vi "Labview_code_used_to_design_external_transceiver.vi"() -> ()   [LabVIEW 2018]
doc: "Example: Stream to Disk\n\nRecommended Input Signal: 100kHz, 2Vpp, sine wave\n\nDevices Supported: Refer to NI Example Finder\n\nLabVIEW Description:\n\nThis example demonstrates streaming a continuous acquisition to disk. It configures and starts one acquisition that is never triggered. This is accomplished by configuring a software trigger and never sending the software trigger. Therefore, the digitizer will continuously acquire data into its onboard memory until Abort or Close is called. \n\nThe loop continuously fetches data from onboard memory and streams it to a binary file. If the sampling rate is low, the computer can fetch all the data from the digitizer, so data is never overwritten. However, at faster sampling rates, the computer will not be able to fetch the data before it is overwritten by new data. This results in the \"data overwritten\" error.\n\nThe input parameters to the Fetch VI include the maximum waveform size to fetch. Since a timeout of zero is set, the digitizer will return however many points are currently available rather than waiting for the requested number of samples. The Fetch VI will return a waveform with the actual number of points fetched. \n\nThe \"relative to\" property determines which samples to fetch from memory. In this example, it is set to the read pointer, which starts at the beginning of the acquisition and is incremented by the actual number of points during each fetch."
uses:
  Control 1.ctl
  <vilib>/Utility/error.llb/DialogType.ctl
  <instrlib>/niScope/Controls/niScope input clock source.ctl
  <instrlib>/niScope/Controls/niScope exportable signals.ctl
  <instrlib>/niScope/Controls/niScope export destinations.ctl
  <instrlib>/niScope/Controls/niScope trigger source digital.ctl
  <vilib>/Analysis/3filter.llb/Filter Passband Type.ctl
  <vilib>/DAQmx/write.llb/DAQmx Write (Digital Wfm 1Chan NSamp).vi
  <vilib>/DAQmx/create/channels.llb/DAQmx Create Channel (DO-Digital Output).vi
  <instrlib>/niScope/Configure/Trigger/niScope Configure Trigger Digital.vi
  <vilib>/DAQmx/configure/timing.llb/DAQmx Timing (Sample Clock).vi
  <vilib>/DAQmx/configure/trigger.llb/DAQmx Start Trigger (Digital Edge).vi
  <vilib>/Waveform/DWDTOps.llb/DWDT Boolean Array to Digital.vi
  <vilib>/Waveform/DWDTOps.llb/DWDT Append Digital Signals.vi
  <vilib>/Waveform/DWDTOps.llb/DWDT Uncompress Digital.vi
  <vilib>/DAQmx/miscellaneous.llb/DAQmx Fill In Error Info.vi
  <instrlib>/niScope/Acquire/Fetch/niScope Fetch Binary 16.vi
  <vilib>/Analysis/3filter.llb/Butterworth Filter (DBL).vi
  <vilib>/measure/maresamp.llb/Resample Waveform (single shot).vi
  <vilib>/Analysis/3filter.llb/FIR Filter (DBL).vi
  <resource>/objmgr/daqmx.rc
  <vilib>/measure/NI_MAPro.lvlib
  <vilib>/Analysis/NI_AAL_SigProc.lvlib
  <vilib>/Analysis/NI_AALBase.lvlib
panel:
  out "x-y":i32
  out "Mod. depth":dbl
  out "Threshold 2":dbl
  out "Threshold 1":dbl
  out "index of element 2":i32
  out "index of element":i32
  out "Peak - Valley":dbl[](graph) caption="Peak - Valley vs. Sample Number"
  out "# of peaks":i32
  out "Resampled data":waveform(dbl)(graph) caption="Signal vs. Time"
  out "Peak det. output":bool[](array[boolean])
  in  "Sample rate":dbl=2000000.0 caption="Digital Output Frequency" step=1000000.0 format="%.3p"
  out "Acquisition Complete":bool=TRUE
  out "Digital Waveform":digitalwaveform(graph)
  in  "Line(s)":tag="PXI1Slot5/port0/line1:3"
  in  "stop":bool
  out "Total Acquired Data (bytes)":i64 format="%.0p"
  in  "Total Samples to Acquire":u64=10000000 step=1048576 format="%.3p"
  in  "Continues data acquisition":bool=TRUE caption="Plot Data?"
  out "Memory per Channel":dbl format="%#_4p"
  out "Measurement Time (min)":dbl format="%.2f"
  out "Samples Used Onboard Memory":dbl(slide)=3898016.0 scale=-1.0..33554432.0 scale format="%.1p"
  out "Status":string="Acquisition in progress."
  out "Actual sample rate":dbl caption="Actual Sample Rate" format="%.3p"
  in  "Enforce realtime":bool=TRUE caption="Enforce Realtime"
  in  "Input Impedance":u32(ring) items=["1 mega ohm", "75 ohms", "50 ohms"]
  in  "Channel BW":T1=5000000.0 format="%.1p"
  in  "Channel":string="0" caption="Channel Name(s)"
  out "Format":string
  in  "Confirm File Replace?":bool
  in  "File path":path=path "C:/Users/trial.txt"
  out "error out":errorcluster {"code" format="%.0x"}
  out "Last Points Fetched":i32=50000 format="%.3p"
  out "Total Points Fetched":i64 format="%.0p"
  in  "resource name":refnum<k15>="PXI1Slot3" caption="Resource Name"
  in  "Max Points Per Fetch":u32=55000 format="%.3p"
  in  "Min sample rate":dbl=20000000.0 caption="Min Sample Rate" step=1000000.0 format="%.3p"
  in  "vertical range":dbl=2.4 caption="Vertical Range" format="%.2f"
  # "Vertical and Horizontal"
  # "Settings"
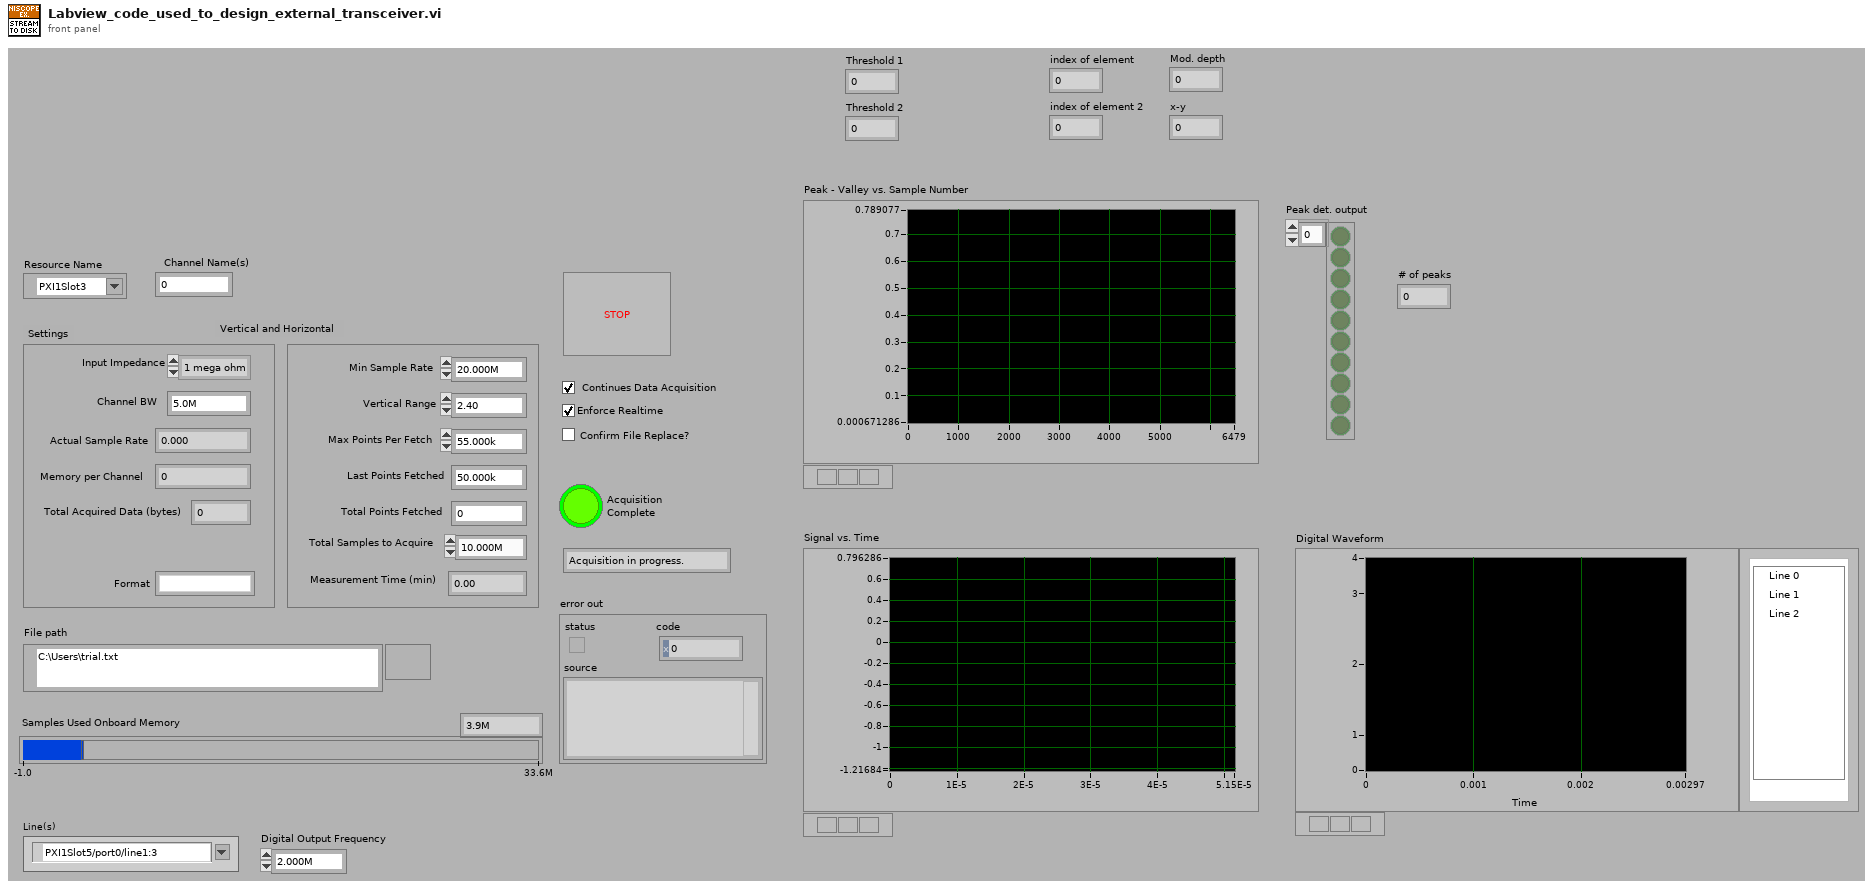
[diagram p1: front panel]
types:
  T1 = typedef "Control 1.ctl" = dbl
  T2 = typedef "niScope trigger source digital.ctl" = string
  T3 = typedef "niScope export destinations.ctl" = string
  T4 = typedef "niScope exportable signals.ctl" = u16
  T5 = typedef "niScope input clock source.ctl" = u16
  T6 = typedef "DialogType.ctl" = u16
  T7 = enum16{"open", "open or create", "create or replace", "create", "open (read only)"}
  T8 = typedef "NI_AALBase.lvlib/Filter Passband Type.ctl" = enum32{"Lowpass", "Highpass", "Bandpass", "Bandstop"}
  T9 = cluster{"alias rejection (dB)":dbl, "normalized bandwidth":dbl}
  T10 = cluster{"actualSamples":i32, "absoluteInitialX":dbl, "relativeInitialX":dbl, "xIncrement":dbl, "offset":dbl, "gain":dbl, "reserved1":dbl, "reserved2":dbl}
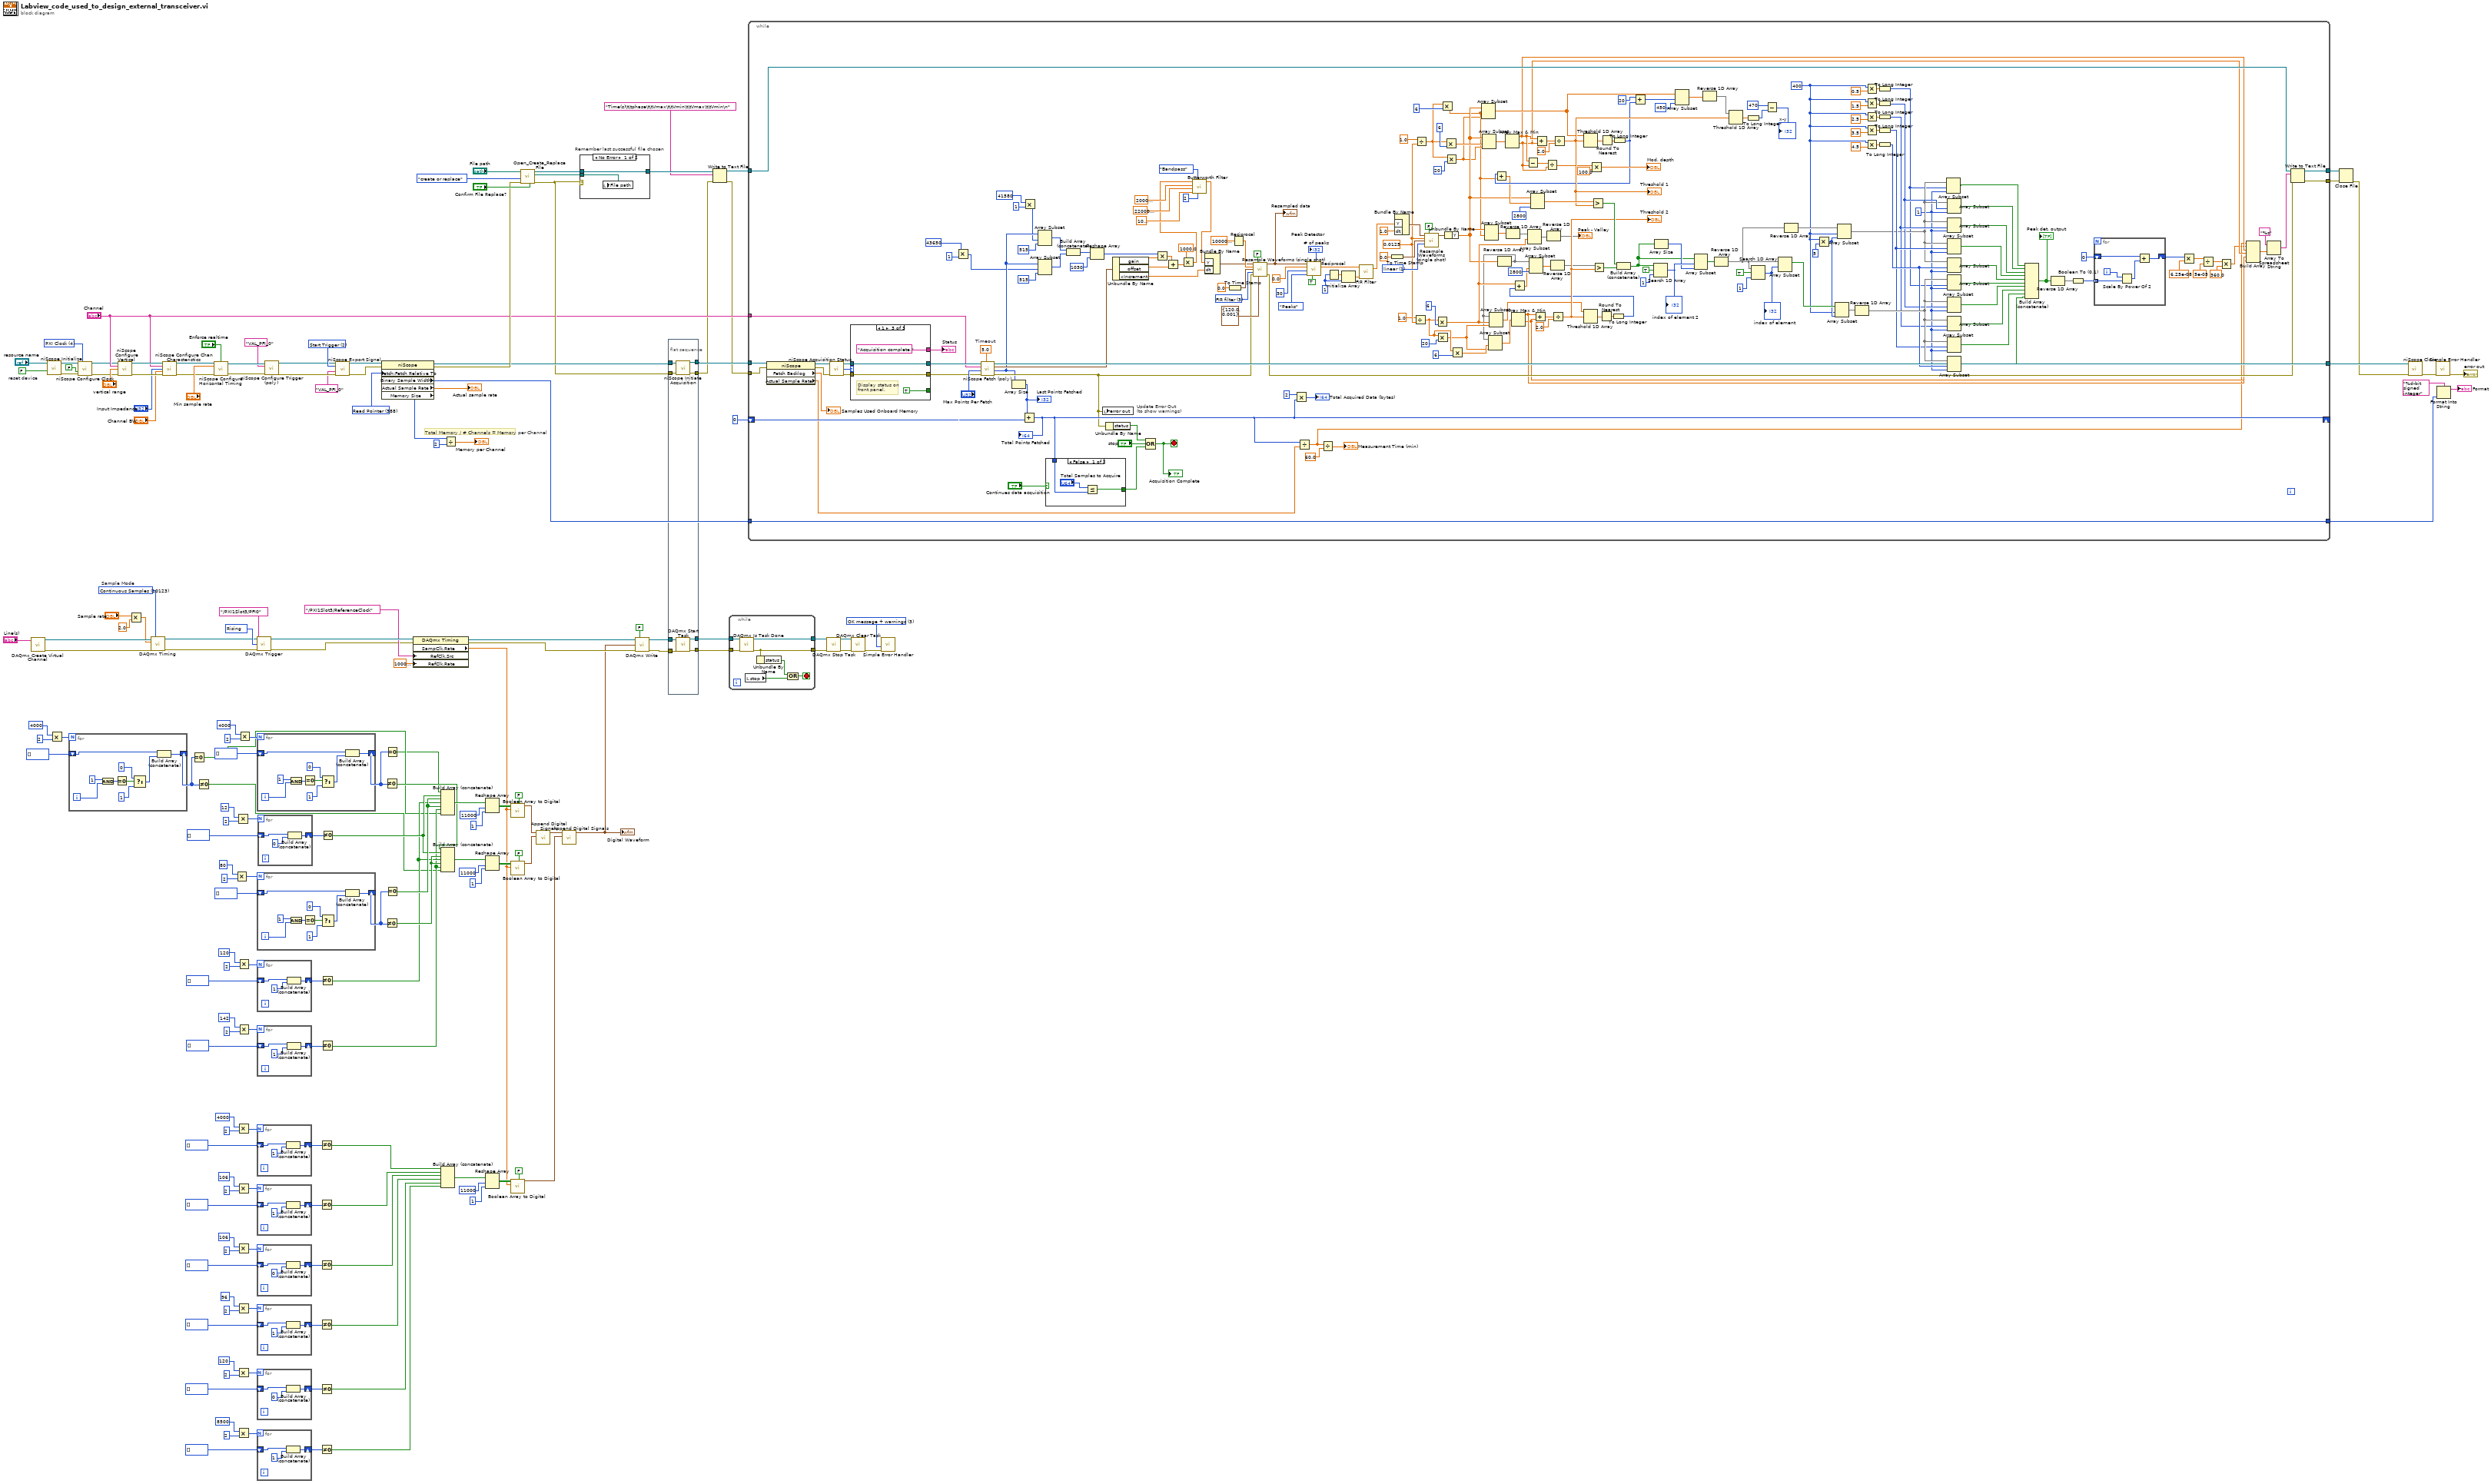
[diagram p0: block diagram]
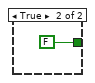
[diagram p3: hidden frame]
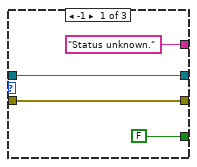
[diagram p4: hidden frame]
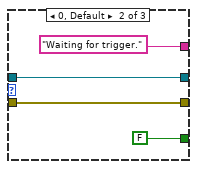
[diagram p5: hidden frame]
diagram:
  w132 = 10280 items=["Rising"=10280, "Falling"=10171] ("edge")
  w137 = T4 2 items=["None"=0, "Start Trigger"=2, "Advance Trigger"=5, "Reference Trigger"=1, "End of Record Event"=4, "End of Acquisition Event"=3, "Ready for Start Event"=7, "Ready for Advance Event"=6, "Ready for Reference Event"=10, "Reference Clock"=100, "Sample Clock"=101, "5 Volt Power"=13] ("signal")
  w142 = 10123 items=["Finite Samples"=10178, "Continuous Samples"=10123, "Hardware Timed Single Point"=12522]  # Sample Mode
  w143 = T5 4 items=["None"=0, "RTSI Clock"=1, "PFI 0"=6, "PFI 1"=2, "PFI 2"=3, "PXI Clock"=4, "External"=5, "Clock In"=7] ("input clock source")
  w151 = T6 3 items=["no dialog", "OK message", "continue or stop message", "OK message + warnings", "continue/stop + warnings"] ("type of dialog (OK msg:1)")
  w163 = 388 items=["Start"=482, "Trigger"=483, "Pretrigger"=477, "Now"=481, "Read Pointer"=388] ("Fetch:Fetch Relative To")
  w181 = FALSE  # reset device
  # "Total Memory / # Channels = Memory per Channel"
  # "Remember last successful file chosen"
  n1 = call-poly <vilib>:"DAQmx Create Virtual Channel.vi"("lines"="Line(s)") -> ("task out"=w66:refnum<k21>, "error out"=w65:errorcluster)  [unwired: 13 in]
  n2 = call <instrlib>:"niScope Initialize.vi"("resource name"="resource name", "reset device"=w181) -> ("instrument handle"=w150:refnum<k15>, "error out"=w149:errorcluster)  [unwired: 12 in]
  n3 = Multiply(x=4000, y=2) -> (x*y=w8:i32)
  n4 = for {
    N: w8 -> [_]
    shift-right: [w189] -> w3
    shift-left: i32[] [] -> [w190]
    i -> [w186]
    n5 = And(x=1, y=w186) -> (x .and. y?=w187:i32)
    n6 = Equal To 0?(x=w187) -> (x = 0?=w185:bool)
    n7 = Select(t=0, s=w185, f=1) -> (s? t:f=w182:i32)
    n8 = Build Array (concatenate)(w190, w182) -> (w189:i32[])
  }
  n9 = call <instrlib>:"niScope Configure Clock.vi"("instrument handle"=w150, "input clock source"=w143, "master enabled"=FALSE, "error in"=w149) -> ("instrument handle out"=w72:refnum<k15>, "error out"=w71:errorcluster)  [unwired: 10 in]
  n10 = call <instrlib>:"niScope Configure Vertical.vi"("instrument handle"=w72, "channels"="Channel", "vertical range"="vertical range", "error in"=w71) -> ("instrument handle out"=w168:refnum<k15>, "error out"=w167:errorcluster)  [unwired: 10 in]
  n11 = Multiply(x="Sample rate", y=2.0) -> (x*y=w63:dbl)
  n12 = call-poly <vilib>:"DAQmx Timing.vi"("task/channels in"=w66, "sample mode"=w142, "rate"=w63, "error in"=w65) -> ("task out"=w130:refnum<k21>, "error out"=w129:errorcluster)  [unwired: 10 in]
  n13 = call <instrlib>:"niScope Configure Chan Characteristics.vi"("instrument handle"=w168, "channels"="Channel", "input impedance"="Input Impedance", "maximum input frequency"="Channel BW", "error in"=w167) -> ("instrument handle out"=w68:refnum<k15>, "error out"=w67:errorcluster)  [unwired: 9 out]
  n14 = Equal To 0?(x=w3) -> (x = 0?=w2:bool[])
  n15 = Not Equal To 0?(x=w3) -> (x != 0?=w5:bool[])
  n16 = call <instrlib>:"niScope Configure Horizontal Timing.vi"("instrument handle"=w68, "enforce realtime"="Enforce realtime", "min sample rate"="Min sample rate", "error in"=w67) -> ("instrument handle out"=w135:refnum<k15>, "error out"=w134:errorcluster)  [unwired: 10 in]
  n17 = Multiply(x=80, y=2) -> (x*y=w92:i32)
  n18 = Multiply(x=12, y=2) -> (x*y=w95:i32)
  n19 = Multiply(x=4000, y=2) -> (x*y=w50:i32)
  n20 = Multiply(x=106, y=2) -> (x*y=w45:i32)
  n21 = Multiply(x=106, y=2) -> (x*y=w40:i32)
  n22 = Multiply(x=96, y=2) -> (x*y=w35:i32)
  n23 = Multiply(x=120, y=2) -> (x*y=w19:i32)
  n24 = Multiply(x=8500, y=2) -> (x*y=w12:i32)
  n25 = Multiply(x=120, y=2) -> (x*y=w89:i32)
  n26 = Multiply(x=142, y=2) -> (x*y=w24:i32)
  n27 = Multiply(x=4000, y=2) -> (x*y=w100:i32)
  n28 = call-poly <vilib>:"DAQmx Trigger.vi"("task/channels in"=w130, "source"=tag "/PXI1Slot3/PFI0", "edge"=w132, "error in"=w129) -> ("task out"=w128:refnum<k21>, "error out"=w69:errorcluster)  [unwired: 10 in]
  n29 = for {
    N: w50 -> [_]
    shift-right: [w191] -> w53
    shift-left: i32[] [] -> [w193]
    n30 = Build Array (concatenate)(w193, 1 ("element")) -> (w191:i32[])
  }
  n31 = for {
    N: w45 -> [_]
    shift-right: [w194] -> w48
    shift-left: i32[] [] -> [w196]
    n32 = Build Array (concatenate)(w196, 1 ("element")) -> (w194:i32[])
  }
  n33 = for {
    N: w40 -> [_]
    shift-right: [w197] -> w43
    shift-left: i32[] [] -> [w199]
    n34 = Build Array (concatenate)(w199, 0 ("element")) -> (w197:i32[])
  }
  n35 = for {
    N: w35 -> [_]
    shift-right: [w200] -> w38
    shift-left: i32[] [] -> [w202]
    n36 = Build Array (concatenate)(w202, 1 ("element")) -> (w200:i32[])
  }
  n37 = for {
    N: w19 -> [_]
    shift-right: [w203] -> w21
    shift-left: i32[] [] -> [w205]
    n38 = Build Array (concatenate)(w205, 0 ("element")) -> (w203:i32[])
  }
  n39 = for {
    N: w12 -> [_]
    shift-right: [w206] -> w15
    shift-left: i32[] [] -> [w208]
    n40 = Build Array (concatenate)(w208, 1 ("element")) -> (w206:i32[])
  }
  n41 = for {
    N: w100 -> [_]
    shift-right: [w216] -> w107
    shift-left: i32[] [] -> [w217]
    i -> [w213]
    n42 = And(x=1, y=w213) -> (x .and. y?=w214:i32)
    n43 = Equal To 0?(x=w214) -> (x = 0?=w212:bool)
    n44 = Select(t=0, s=w212, f=1) -> (s? t:f=w209:i32)
    n45 = Build Array (concatenate)(w217, w209) -> (w216:i32[])
  }
  n46 = for {
    N: w92 -> [_]
    shift-right: [w225] -> w105
    shift-left: i32[] [] -> [w226]
    i -> [w222]
    n47 = And(x=1, y=w222) -> (x .and. y?=w223:i32)
    n48 = Equal To 0?(x=w223) -> (x = 0?=w221:bool)
    n49 = Select(t=0, s=w221, f=1) -> (s? t:f=w218:i32)
    n50 = Build Array (concatenate)(w226, w218) -> (w225:i32[])
  }
  n51 = for {
    N: w89 -> [_]
    shift-right: [w227] -> w101
    shift-left: i32[] [] -> [w229]
    n52 = Build Array (concatenate)(w229, 1 ("element")) -> (w227:i32[])
  }
  n53 = for {
    N: w24 -> [_]
    shift-right: [w230] -> w27
    shift-left: i32[] [] -> [w232]
    n54 = Build Array (concatenate)(w232, 1 ("element")) -> (w230:i32[])
  }
  n55 = for {
    N: w95 -> [_]
    shift-right: [w233] -> w103
    shift-left: i32[] [] -> [w235]
    n56 = Build Array (concatenate)(w235, 0 ("element")) -> (w233:i32[])
  }
  n57 = call-poly <instrlib>:"niScope Configure Trigger (poly).vi"("instrument handle"=w135, "trigger source"=T2 "VAL_PFI_0", "error in"=w134) -> ("instrument handle out"=w118:refnum<k15>, "error out"=w138:errorcluster)  [unwired: 11 in]
  n58 = Not Equal To 0?(x=w53) -> (x != 0?=w31:bool[])
  n59 = Not Equal To 0?(x=w48) -> (x != 0?=w34:bool[])
  n60 = Not Equal To 0?(x=w43) -> (x != 0?=w32:bool[])
  n61 = Not Equal To 0?(x=w38) -> (x != 0?=w33:bool[])
  n62 = Not Equal To 0?(x=w21) -> (x != 0?=w17:bool[])
  n63 = Not Equal To 0?(x=w15) -> (x != 0?=w11:bool[])
  n64 = Not Equal To 0?(x=w101) -> (x != 0?=w81:bool[])
  n65 = Not Equal To 0?(x=w27) -> (x != 0?=w23:bool[])
  n66 = Not Equal To 0?(x=w103) -> (x != 0?=w83:bool[])
  n67 = call <instrlib>:"niScope Export Signal.vi"("instrument handle"=w118, "signal"=w137, "output terminal"=T3 "VAL_PFI_0", "error in"=w138) -> ("instrument handle out"=w119:refnum<k15>, "error out"=w117:errorcluster)  [unwired: 10 in]
  n68 = property class="niScope"(reference=w119, error in=w117, "Fetch:Fetch Relative To"=w163) -> (reference out=w125:refnum<k15>, error out=w161:errorcluster, "Binary Sample Width"=w158:i32, "Actual Sample Rate"=→"Actual sample rate":dbl, "Memory Size"=w159:i32)
  n69 = Not Equal To 0?(x=w107) -> (x != 0?=w4:bool[])
  n70 = Not Equal To 0?(x=w105) -> (x != 0?=w82:bool[])
  n71 = Equal To 0?(x=w107) -> (x = 0?=w1:bool[])
  n72 = Equal To 0?(x=w105) -> (x = 0?=w84:bool[])
  n73 = property class="DAQmx Timing"(reference=w128, error in=w69, "RefClk.Src"=tag "/PXI1Slot3/ReferenceClock" ("source"), "RefClk.Rate"=10000000.0 ("SampClk.Timebase.Rate")) -> (reference out=w127:refnum<k21>, error out=w126:errorcluster, "SampClk.Rate"=w30:dbl)
  n74 = Build Array (concatenate)(w1, w83, w84, w81, w84, w23, w2) -> (w73:bool[])
  n75 = Build Array (concatenate)(w4, w83, w82, w81, w82, w23, w5) -> (w78:bool[])
  n76 = Build Array (concatenate)(w31, w34, w32, w33, w17, w11) -> (w59:bool[])
  n77 = Divide(x=w159, y=2) -> (x/y=→"Memory per Channel":dbl)
  n78 = Reshape Array(w73, 11000 ("dimension size"), 1 ("dimension size")) -> (w85:bool[][])
  n79 = Reshape Array(w78, 11000 ("dimension size"), 1 ("dimension size")) -> (w76:bool[][])
  n80 = Reshape Array(w59, 11000 ("dimension size"), 1 ("dimension size")) -> (w57:bool[][])
  n81 = call-poly <vilib>:"Boolean Array to Digital.vi"("compress data (F)"=FALSE, "sample rate"=w30, "boolean array"=w85) -> ("digital waveform"=w75:digitalwaveform)  [unwired: 7 in, 1 out]
  n82 = call-poly <vilib>:"Boolean Array to Digital.vi"("compress data (F)"=FALSE, "sample rate"=w30, "boolean array"=w76) -> ("digital waveform"=w74:digitalwaveform)  [unwired: 7 in, 1 out]
  n83 = call-poly <vilib>:"Boolean Array to Digital.vi"("compress data (F)"=FALSE, "sample rate"=w30, "boolean array"=w57) -> ("digital waveform"=w55:digitalwaveform)  [unwired: 7 in, 1 out]
  n84 = call <vilib>:"Open_Create_Replace File.vi"("advisory dialog? (display:T)"="Confirm File Replace?", "error in (no error)"=w161, "function (open:0)"=T7."create or replace", "file path"="File path") -> ("error out"=w124:errorcluster, "new file path"=w176:path, "refnum"=w177:refnum<file>)  [unwired: 4 in, 1 out]
  n85 = call-poly <vilib>:"Append Digital Signals.vi"("digital waveform (low bits)"=w74, "digital waveform (high bits)"=w75) -> ("digital waveform out"=w56:digitalwaveform)  [unwired: 8 in, 1 out]
  n86 = call-poly <vilib>:"Append Digital Signals.vi"("digital waveform (low bits)"=w55, "digital waveform (high bits)"=w56) -> ("digital waveform out"=w29:digitalwaveform)  [unwired: 8 in, 1 out]
  "Digital Waveform" <- w29
  n87 = case shown="No Error" w124 {
    tunnel: w176 -> [w236 _]
    tunnel: w177 -> [w237 w238]
    tunnel: [w237 w238] -> w114
    frame No Error {
      n88 = local write "File path"(w236) -> ()
    }
    frame Error {
    }
  }
  n89 = call-poly <vilib>:"DAQmx Write.vi"("task/channels in"=w127, "auto start"=FALSE, "data"=w29, "error in"=w126) -> ("task out"=w148:refnum<k21>, "error out"=w147:errorcluster)  [unwired: 9 in, 1 out]
  n90 = flat-sequence {
    tunnel: w148 -> [w246]
    tunnel: w147 -> [w245]
    tunnel: w125 -> [w242]
    tunnel: w124 -> [w241]
    tunnel: [w244] -> w116
    tunnel: [w243] -> w115
    tunnel: [w240] -> w123
    tunnel: [w239] -> w110
    frame #0 {
      n91 = call <instrlib>:"niScope Initiate Acquisition.vi"("instrument handle"=w242, "error in"=w241) -> ("instrument handle out"=w240:refnum<k15>, "error out"=w239:errorcluster)  [unwired: 12 in]
      n92 = call <vilib>:"DAQmx Start Task.vi"("task/channels in"=w246, "error in"=w245) -> ("task out"=w244:refnum<k21>, "error out"=w243:errorcluster)  [unwired: 12 in]
    }
  }
  n93 = Write to Text File(file (use dialog)=w114, text="Time(s)\t\tphase\t\tVmax\t\tVmin\t\tVmax\t\tVmin\n", error in=w110) -> (refnum out=w10:refnum<file>, error out=w109:errorcluster)  [unwired: 1 in, 1 out]
  n94 = while {
    tunnel: [w253] -> w146
    tunnel: [w252] -> w145
    tunnel: w116 -> [w248]
    tunnel: w115 -> [w247]
    stop <- w251 stop-if-true
    n95 = call <vilib>:"DAQmx Is Task Done.vi"("task/channels in"=w248, "error in"=w247) -> ("task out"=w253:refnum<k21>, "error out"=w252:errorcluster)  [unwired: 11 in, 1 out]
    n96 = local read "stop"() -> (w250:bool)
    n97 = Unbundle By Name(w252) -> ("status"=w249:bool)
    n98 = Compound Arithmetic op=OR(w249, w250) -> (w251:bool)
  }
  n99 = while {
    shift-left: 0 -> [w465]
    shift-right: [w445] -> _
    tunnel: "Channel" -> [w449]
    tunnel: w158 -> [w462]
    tunnel: [w462] -> w171
    tunnel: [w460] -> w169
    tunnel: w123 -> [w441]
    tunnel: w109 -> [w440]
    tunnel: [w421] -> w113
    tunnel: [w401] -> w111
    tunnel: w10 -> [w356]
    stop <- w438 stop-if-true
    w260 = 400 ("length")
    w301 = 1 ("x")
    w295 = 1 ("length")
    w391 = u16 1 items=["coerce", "linear", "spline", "FIR filter"] ("interpolation mode")
    w350 = 0.0125 ("dt")
    w418 = u16 3 items=["coerce", "linear", "spline", "FIR filter"] ("interpolation mode")
    w463 = 5.0  # Timeout
    # "Update Error Out\n(to show warnings)"
    n100 = property class="niScope"(reference=w441, error in=w440) -> (reference out=w411:refnum<k15>, error out=w442:errorcluster, "Fetch Backlog"=→"Samples Used Onboard Memory":dbl, "Actual Sample Rate"=w450:dbl)
    n101 = call <instrlib>:"niScope Acquisition Status.vi"("instrument handle"=w411, "error in"=w442) -> ("instrument handle out"=w457:refnum<k15>, "acquisition status"=w459:i32, "error out"=w458:errorcluster)  [unwired: 11 out]
    n102 = case shown="1" w459 {
      tunnel: w458 -> [w475 w480 w484]
      tunnel: w457 -> [w476 w481 w485]
      tunnel: ["Status unknown." "Waiting for trigger." "Acquisition complete."] -> w456
      tunnel: [w476 w481 w485] -> w454
      tunnel: [w475 w480 w484] -> w455
      tunnel: [FALSE ("value") FALSE ("value") TRUE ("value")] -> _
      frame -1 {
      }
      frame 0, Default {
      }
      frame 1 {
        # "Display status on\nfront panel."
      }
    }
    "Status" <- w456
    n103 = Multiply(x=43650 ("index"), y=1) -> (x*y=w362:i32)
    n104 = call-poly <instrlib>:"niScope Fetch (poly).vi"("timeout"=w463, "error in"=w455, "numSamples"="Max Points Per Fetch", "channels"=w449, "instrument handle"=w454) -> ("error out"=w402:errorcluster, "wfm"=w396:i16[], "wfm info"=w432:T10, "instrument handle out"=w460:refnum<k15>)  [unwired: 3 in]
    n105 = Array Size(array=w396) -> (size(s)=w461:i32)
    "Last Points Fetched" <- w461
    n106 = Add(x=w461, y=w465) -> (x+y=w445:i32)
    "Total Points Fetched" <- w445
    n107 = Multiply(x=41580 ("index"), y=1) -> (x*y=w365:i32)
    n108 = Array Subset(array=w396, index=w365, length=515) -> (w424:i16[])
    n109 = Array Subset(array=w396, index=w362, length=515) -> (w425:i16[])
    n110 = case shown="False" "Continues data acquisition" {
      tunnel: [w471 FALSE] -> w453
      tunnel: w445 -> [w472 _]
      frame False {
        n111 = Less Or Equal?(x="Total Samples to Acquire", y=w472) -> (x <= y?=w471:bool)
      }
      frame True {
      }
    }
    n112 = Build Array (concatenate)(w424, w425) -> (w423:i16[])
    n113 = Reshape Array(w423, 1030 ("dimension size")) -> (w395:i16[])
    n114 = local write "error out"(w402) -> ()
    n115 = Unbundle By Name(w402) -> ("status"=w439:bool)
    n116 = Unbundle By Name(w432) -> ("gain"=w435:dbl, "offset"=w436:dbl, "xIncrement"=w412:dbl)
    n117 = Compound Arithmetic op=OR(w439, "stop", w453) -> (w438:bool)
    "Acquisition Complete" <- w438
    n118 = Multiply(x=w395, y=w435) -> (x*y=w437:dbl[])
    n119 = Add(x=w437, y=w436) -> (x+y=w434:dbl[])
    n120 = Multiply(x=1000.0, y=w434) -> (x*y=w304:dbl[])
    n121 = call-poly <vilib>:"Butterworth Filter.vi"("order"=2, "filter type"=Filter_Passband_Type."Bandpass", "low cutoff freq: fl"=1000000.0, "high cutoff freq: fh"=2200000.0, "sampling freq: fs"=20000000.0, "X"=w304) -> ("Filtered X"=w303:dbl[])  [unwired: 2 in, 1 out]
    n122 = Bundle By Name("Y"=w303, "dt"=w412) -> (w360:waveform(dbl))  [unwired: 1 in]
    n123 = To Time Stamp(1:0.0 ("number")) -> (0:w415:timestamp)
    n124 = Reciprocal(x=100000000.0) -> (1/x=w417:dbl)
    n125 = call-poly <vilib>:"Resample Waveforms (single shot).vi"("waveform in"=w360, "open interval? (F)"=FALSE, "dt"=w417, "t0"=w415, "interpolation mode"=w418, "error in (no error)"=w402, "FIR filter specifications"=T9 {"alias rejection (dB)"=120.0, "normalized bandwidth"=0.001}) -> ("resampled waveform out"=w359:waveform(dbl), "error out"=w379:errorcluster)  [unwired: 5 in, 2 out]
    "Resampled data" <- w359
    n126 = Multiply(x=u64 2, y=w445) -> (x*y=→"Total Acquired Data (bytes)":u64)
    n127 = Divide(x=w445, y=w450) -> (x/y=w255:dbl)
    n128 = call <vilib>:"Peak Detector.vi"("initialize (T)"=TRUE, "peaks/valleys"=enum32{"Peaks", "Valleys"}."Peaks" ("peaks/valleys 2"), "width"=30, "threshold"=0.0, "X"=w359) -> ("Amplitudes"=w298:dbl[], "# found"=→"# of peaks":i32)  [unwired: 2 in, 3 out]
    n129 = Divide(x=w255, y=60.0) -> (x/y=→"Measurement Time (min)":dbl)
    n130 = Reciprocal(x=w301) -> (1/x=w302:dbl)
    n131 = Initialize Array(w302, w301) -> (w300:dbl[])
    n132 = call-poly <vilib>:"FIR Filter.vi"("FIR Coefficients"=w300, "X"=w298) -> ("Filtered X"=w299:dbl[])  [unwired: 2 in, 1 out]
    n133 = To Time Stamp(1:0.0 ("number")) -> (0:w389:timestamp)
    n134 = Bundle By Name("Y"=w299, "dt"=1.0) -> (w393:waveform(dbl))  [unwired: 1 in]
    n135 = Divide(x=1.0, y=w350) -> (x/y=w268:dbl)
    n136 = Divide(x=1.0, y=w350) -> (x/y=w270:dbl)
    n137 = call-poly <vilib>:"Resample Waveforms (single shot).vi"("waveform in"=w393, "open interval? (F)"=FALSE, "dt"=w350, "t0"=w389, "interpolation mode"=w391) -> ("resampled waveform out"=w394:waveform(dbl))  [unwired: 7 in, 3 out]
    n138 = Multiply(x=w268, y=6 ("index")) -> (x*y=w276:dbl)
    n139 = Multiply(x=w268, y=20 ("length")) -> (x*y=w266:dbl)
    n140 = Multiply(x=w270, y=6 ("index")) -> (x*y=w262:dbl)
    n141 = Multiply(x=w270, y=6 ("index")) -> (x*y=w277:dbl)
    n142 = Multiply(x=w270, y=20 ("length")) -> (x*y=w263:dbl)
    n143 = Unbundle By Name(w394) -> ("Y"=w271:dbl[])
    n144 = Multiply(x=w268, y=6 ("length")) -> (x*y=w267:dbl)
    n145 = Array Subset(array=w271, index=w262, length=w263) -> (w273:dbl[])
    n146 = Array Subset(array=w271, index=w277, length=w263) -> (w272:dbl[])
    n147 = Array Subset(array=w271, index=w262) -> (w280:dbl[])  [unwired: 1 in]
    n148 = Reverse 1D Array(array=w271) -> (reversed array=w264:dbl[])
    n149 = Array Subset(array=w264, index=w267, length=w266) -> (w265:dbl[])
    n150 = Array Subset(array=w264, index=w276, length=w266) -> (w290:dbl[])
    n151 = Array Max & Min(array=w272) -> (max value=w259:dbl, min value=w258:dbl)  [unwired: 2 out]
    n152 = Reverse 1D Array(array=w280) -> (reversed array=w279:dbl[])
    n153 = Array Max & Min(array=w265) -> (max value=w257:dbl, min value=w256:dbl)  [unwired: 2 out]
    n154 = Subtract(x=w259, y=w258) -> (x-y=w314:dbl)
    n155 = Array Subset(array=w279, index=w276) -> (w278:dbl[])  [unwired: 1 in]
    n156 = Add(x=w257, y=w256) -> (x+y=w348:dbl)
    n157 = Add(x=w259, y=w258) -> (x+y=w383:dbl)
    n158 = Divide(x=w314, y=w258) -> (x/y=w313:dbl)
    n159 = Reverse 1D Array(array=w278) -> (reversed array=→"Peak - Valley":dbl[])
    n160 = Divide(x=w348, y=2.0) -> (x/y=w315:dbl)
    "Threshold 2" <- w315
    n161 = Divide(x=w383, y=2.0) -> (x/y=w340:dbl)
    "Threshold 1" <- w340
    n162 = Threshold 1D Array(2:w340, 3:w273) -> (0:w281:dbl)  [unwired: 1 in]
    n163 = Threshold 1D Array(2:w315, 3:w290) -> (0:w288:dbl)  [unwired: 1 in]
    n164 = Multiply(x=w313, y=100.0) -> (x*y=→"Mod. depth":dbl)
    n165 = Round To Nearest(number=w288) -> (nearest integer value=w289:dbl)
    n166 = Round To Nearest(number=w281) -> (nearest integer value=w282:dbl)
    n167 = To Long Integer(number=w289) -> (32bit integer=w286:i32)
    n168 = Add(x=w276, y=w286) -> (x+y=w287:dbl)
    n169 = Array Subset(array=w264, index=w287, length=2800) -> (w346:dbl[])
    n170 = Reverse 1D Array(array=w346) -> (reversed array=w310:dbl[])
    n171 = Greater?(x=w310, y=w315) -> (0:w377:bool[])
    n172 = To Long Integer(number=w282) -> (32bit integer=w285:i32)
    n173 = Add(x=w285, y=w262) -> (x+y=w284:dbl)
    n174 = Array Subset(array=w271, index=w284, length=2800) -> (w341:dbl[])
    n175 = Greater?(x=w341, y=w340) -> (0:w378:bool[])
    n176 = Build Array (concatenate)(w378, w377) -> (w345:bool[])
    n177 = Add(x=20, y=w285) -> (x+y=w336:i32)
    n178 = Search 1D Array(1D array=w345, element=TRUE, start index (0)=1) -> (index of element=w430:i32)
    "index of element 2" <- w430
    n179 = Array Size(array=w345) -> (size(s)=w387:i32)
    n180 = Array Subset(array=w273, index=w336, length=450) -> (w335:dbl[])
    n181 = Array Subset(array=w345, index=w430, length=w387) -> (w386:bool[])
    n182 = Reverse 1D Array(array=w335) -> (reversed array=w334:dbl[])
    n183 = Reverse 1D Array(array=w386) -> (reversed array=w357:bool[])
    n184 = Threshold 1D Array(2:w340, 3:w334) -> (0:w339:dbl)  [unwired: 1 in]
    n185 = To Long Integer(number=w339) -> (32bit integer=w283:i32)
    n186 = Search 1D Array(1D array=w357, element=TRUE, start index (0)=1) -> (index of element=w428:i32)
    "index of element" <- w428
    n187 = Subtract(x=470 ("length"), y=w283) -> (x-y=→"x-y":i32)
    n188 = Array Subset(array=w357, index=w428) -> (w358:bool[])  [unwired: 1 in]
    n189 = Reverse 1D Array(array=w357) -> (reversed array=w332:bool[])
    n190 = Multiply(x=w260, y=5) -> (x*y=w330:i32)
    n191 = Array Subset(array=w358, index=w260, length=w330) -> (w384:bool[])
    n192 = Array Subset(array=w332, index=w260, length=w330) -> (w296:bool[])
    n193 = Reverse 1D Array(array=w384) -> (reversed array=w361:bool[])
    n194 = Multiply(x=w260, y=0.5) -> (x*y=w322:dbl)
    n195 = Multiply(x=w260, y=1.5) -> (x*y=w328:dbl)
    n196 = Multiply(x=w260, y=2.5) -> (x*y=w326:dbl)
    n197 = Multiply(x=w260, y=3.5) -> (x*y=w324:dbl)
    n198 = Multiply(x=w260, y=4.5) -> (x*y=w320:dbl)
    n199 = To Long Integer(number=w322) -> (32bit integer=w294:i32)
    n200 = To Long Integer(number=w328) -> (32bit integer=w316:i32)
    n201 = To Long Integer(number=w326) -> (32bit integer=w317:i32)
    n202 = To Long Integer(number=w324) -> (32bit integer=w318:i32)
    n203 = To Long Integer(number=w320) -> (32bit integer=w319:i32)
    n204 = Array Subset(array=w296, index=w294, length=w295) -> (w297:bool[])
    n205 = Array Subset(array=w296, index=w316, length=w295) -> (w376:bool[])
    n206 = Array Subset(array=w296, index=w317, length=w295) -> (w375:bool[])
    n207 = Array Subset(array=w296, index=w318, length=w295) -> (w374:bool[])
    n208 = Array Subset(array=w296, index=w319, length=w295) -> (w373:bool[])
    n209 = Array Subset(array=w361, index=w294, length=w295) -> (w372:bool[])
    n210 = Array Subset(array=w361, index=w316, length=w295) -> (w371:bool[])
    n211 = Array Subset(array=w361, index=w317, length=w295) -> (w370:bool[])
    n212 = Array Subset(array=w361, index=w318, length=w295) -> (w369:bool[])
    n213 = Array Subset(array=w361, index=w319, length=w295) -> (w368:bool[])
    n214 = Build Array (concatenate)(w297, w376, w375, w374, w373, w372, w371, w370, w369, w368) -> (w343:bool[])
    "Peak det. output" <- w343
    n215 = Reverse 1D Array(array=w343) -> (reversed array=w344:bool[])
    n216 = Boolean To (0,1)(Boolean=w344) -> (0, 1=w342:i16[])
    n217 = for {
      tunnel: w342 -> [w469] mode=indexing
      shift-right: [w468] -> w404
      shift-left: i16 0 -> [w466]
      i -> [w470]
      n218 = Scale By Power Of 2(n=w470, x=w469) -> (x*2^n=w467:i16)
      n219 = Add(x=w466, y=w467) -> (x+y=w468:i16)
    }
    n220 = Multiply(x=w404, y=6.25e-08) -> (x*y=w408:dbl)
    n221 = Divide(x=w408, y=5e-05) -> (x/y=w406:dbl)
    n222 = Multiply(x=w406, y=360.0) -> (x*y=w254:dbl)
    n223 = Build Array(w255, w254, w259, w258, w257, w256) -> (w420:dbl[])
    n224 = Array To Spreadsheet String(array=w420, 3:"%s" ("format string")) -> (spreadsheet string=w403:string)  [unwired: 1 in]
    n225 = Write to Text File(file (use dialog)=w356, text=w403, error in=w379) -> (refnum out=w421:refnum<file>, error out=w401:errorcluster)  [unwired: 1 in, 1 out]
  }
  n226 = call <vilib>:"DAQmx Stop Task.vi"("task/channels in"=w146, "error in"=w145) -> ("task out"=w153:refnum<k21>, "error out"=w152:errorcluster)  [unwired: 12 in]
  n227 = call <vilib>:"DAQmx Clear Task.vi"("task in"=w153, "error in"=w152) -> ("error out"=w154:errorcluster)  [unwired: 13 in]
  n228 = call <vilib>:"Simple Error Handler.vi"("type of dialog (OK msg:1)"=w151, "error in (no error)"=w154) -> ()  [unwired: 3 in, 5 out]
  n229 = Close File(refnum=w113, error in=w111) -> (error out=w156:errorcluster)  [unwired: 1 out]
  n230 = call <instrlib>:"niScope Close.vi"("instrument handle"=w169, "error in"=w156) -> ("error out"=w157:errorcluster)  [unwired: 13 in]
  n231 = call <vilib>:"Simple Error Handler.vi"("error in (no error)"=w157) -> ("error out"=→"error out":errorcluster)  [unwired: 4 in, 4 out]
  n232 = Format Into String(format string="%d-bit signed integer", w171) -> (resulting string=→"Format":string)  [unwired: 2 in, 1 out]
